vi "ScanFlyCap.vi"() -> ()   [LabVIEW 2022 SP3]
uses:
  <vilib>/userdefined/High Color/IMAQdx.ctl
  <vilib>/Utility/file.llb/Write To Spreadsheet File (DBL).vi
  <vilib>/vision/driver/NI_Vision_Acquisition_Software.lvlib
  <resource>/objmgr/IMAQImage.rc
panel:
  out "Identify":i32
  in  "ActiveFlyCapControl":refnum<k7>(container)
  in  "ExitSendCmd":bool
  out "X":dbl[](array[numeric])
  in  "Tab Control":enum32{"Image", "Scan", "Motors", "Spectra"}(tab)
  out "Camera?":bool
  out "Image":T1(plugin-control)
  out "Remaining Minutes":i32
  out "Progress Bar":dbl(slide) scale=0.0..1.0
  in  "Sample #":u16
  in  "Save Folder":path=path "D:/Scan Test"
  in  "Root File Name":string="Sample"
  out "Cross Plane Length (mm)":sgl=128.0 format="%.3f"
  out "Scan Plane Length (mm)":sgl=128.0 format="%.3f"
  in  "Distance between\nscan lines (mm)":sgl=1.0 min=0.06 max=1000 step=0.06
  in  "Distance between\nplanes (mm)":sgl=1.0 min=0.06 max=1000 step=0.06
  in  "number of planes":u16=1660
  in  "lines per plane":u16=1660 min=1
  out "current plane":u16
  out "current line":u16
  in  "Abort":bool
  in  "start scan":bool
  out "Current File":path
  in  "Axis 2":refnum<k7>(container)
  in  "Axis 1":refnum<k7>(container)
  in  "Home Seq":bool
  in  "Go Home":bool
  out "XY Graph":cluster{"X":dbl[], "Spectral Amplitude":dbl[]}(graph)
  in  "Exposure (*2.375 ms)":u16=2 format="%.3f"
  in  "Display as wavelngth?":bool=TRUE
  in  "Average#":i32=1 min=1
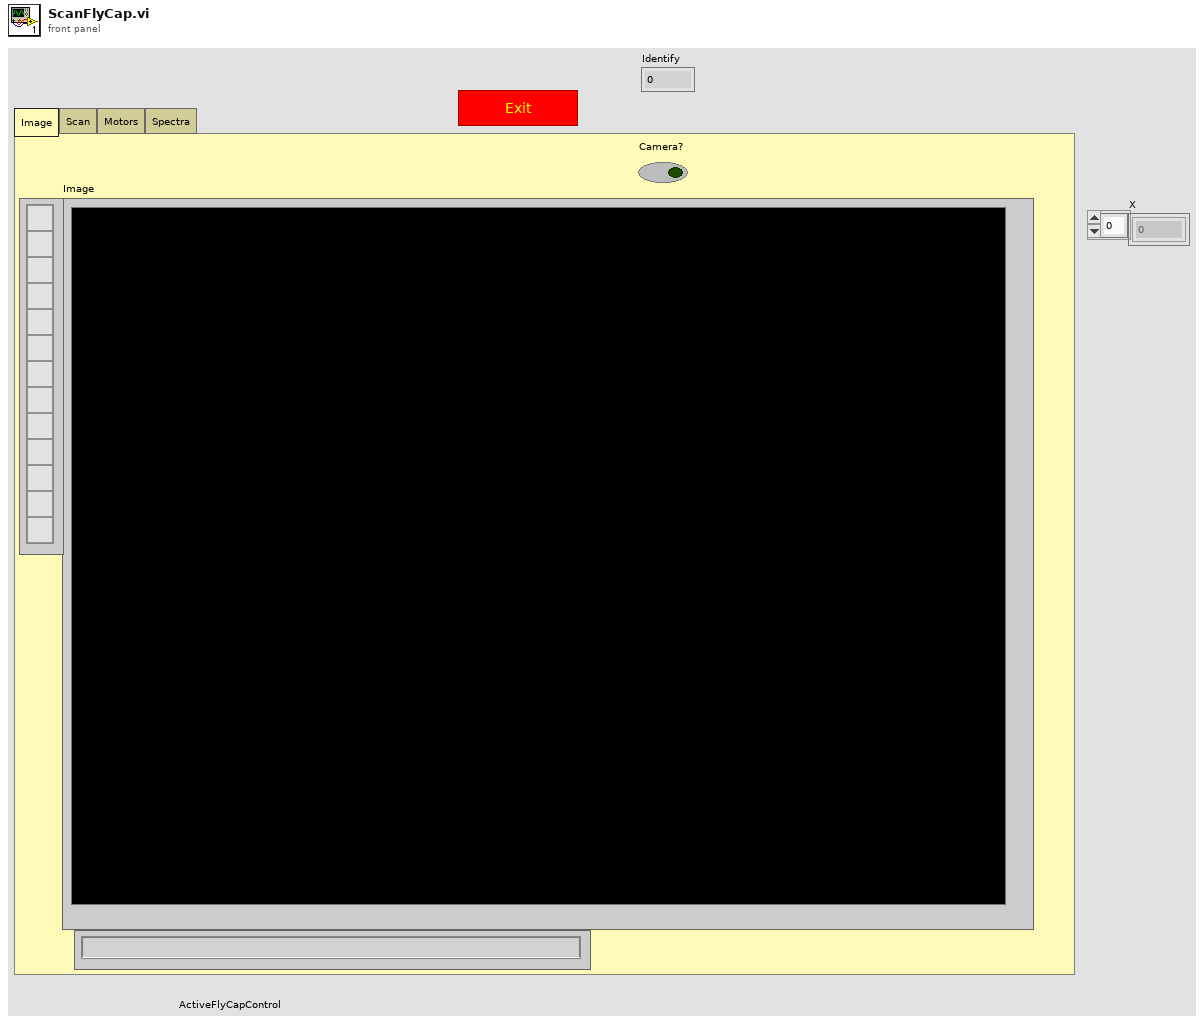
[diagram p1: front panel]
types:
  T1 = typedef "IMAQ Image.ctl" = refnum<image>
  T2 = typedef "Image Type" = u32
  T3 = typedef "IMAQdx.ctl" = refnum<k21>
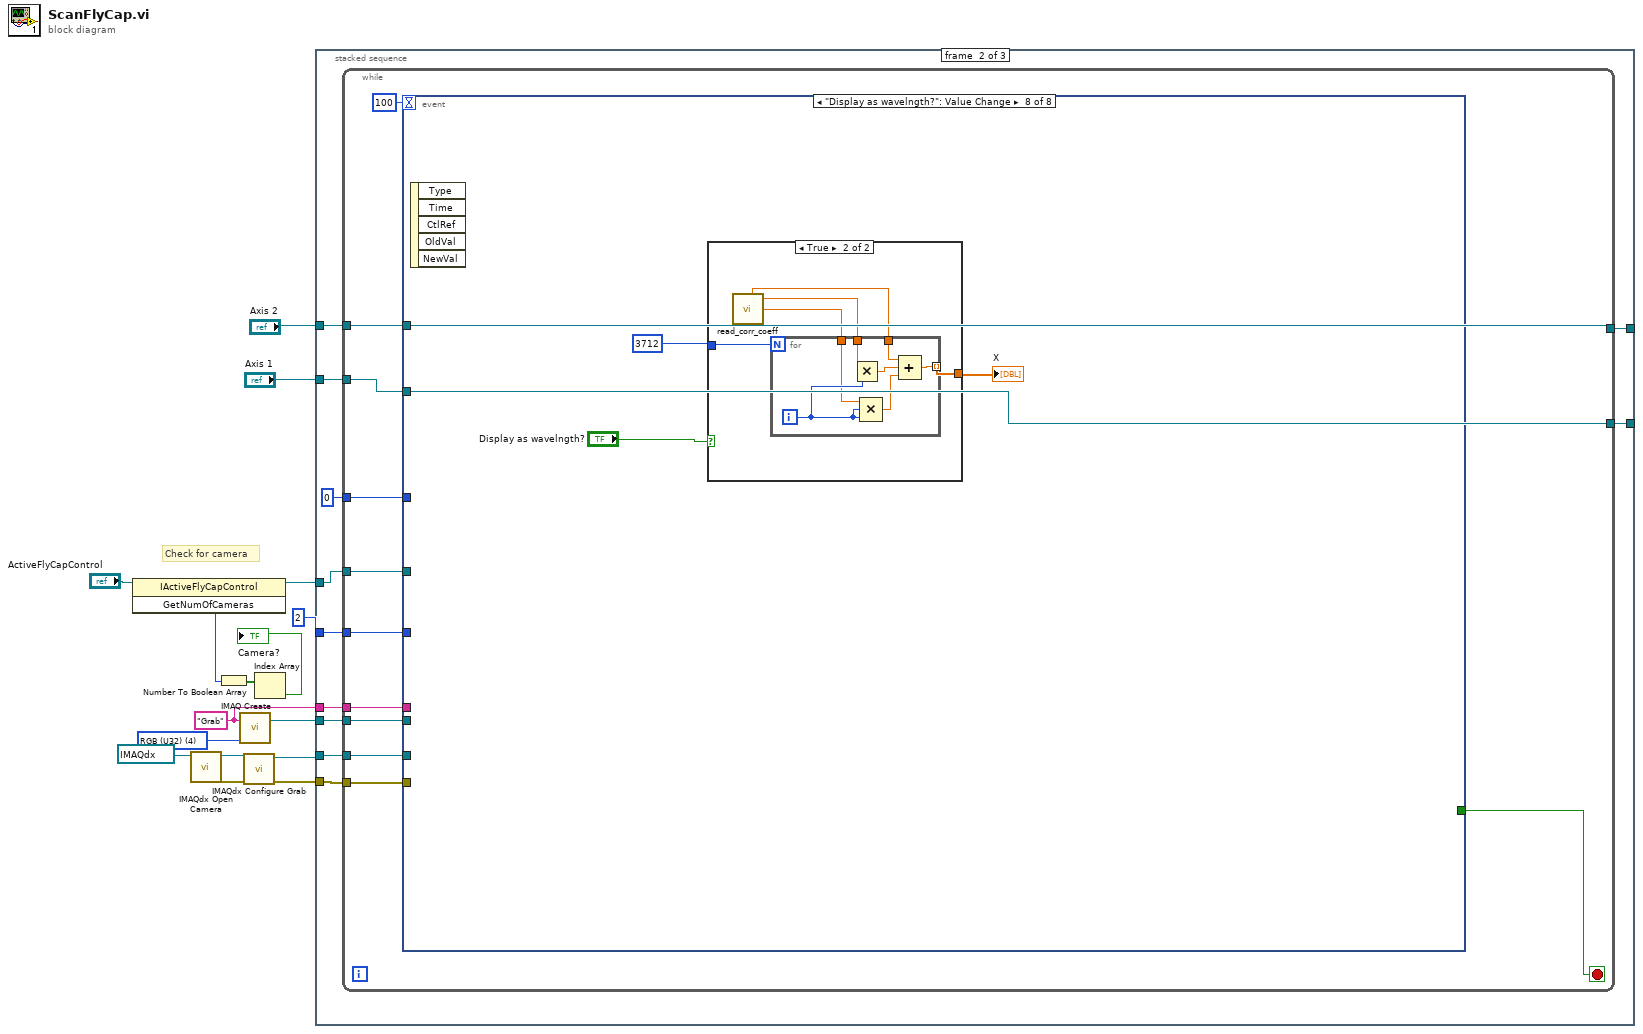
[diagram p0: block diagram]
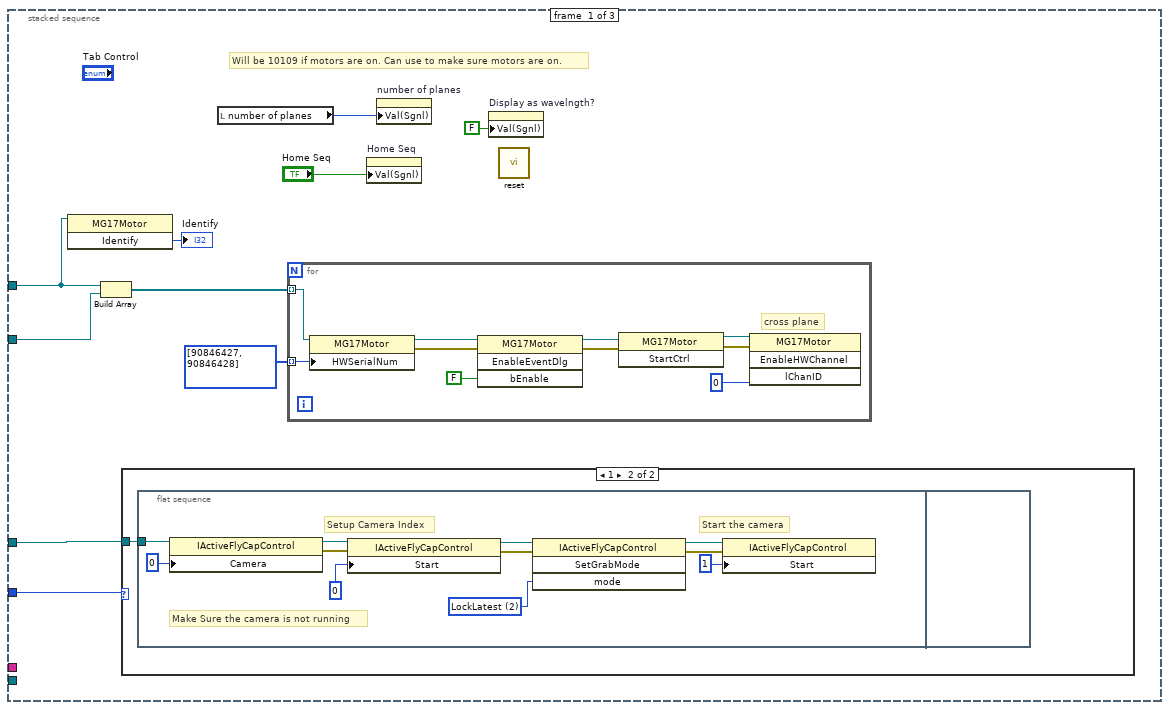
[diagram p2: hidden frame]
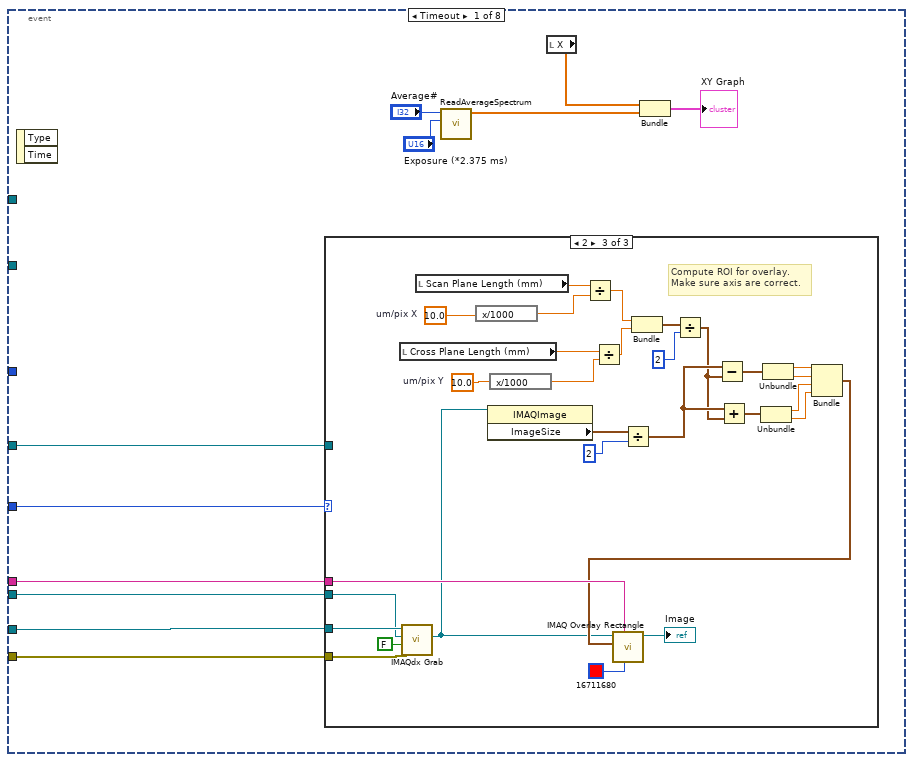
[diagram p4: hidden frame]
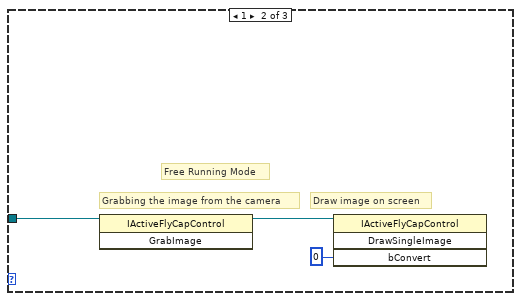
[diagram p6: hidden frame]
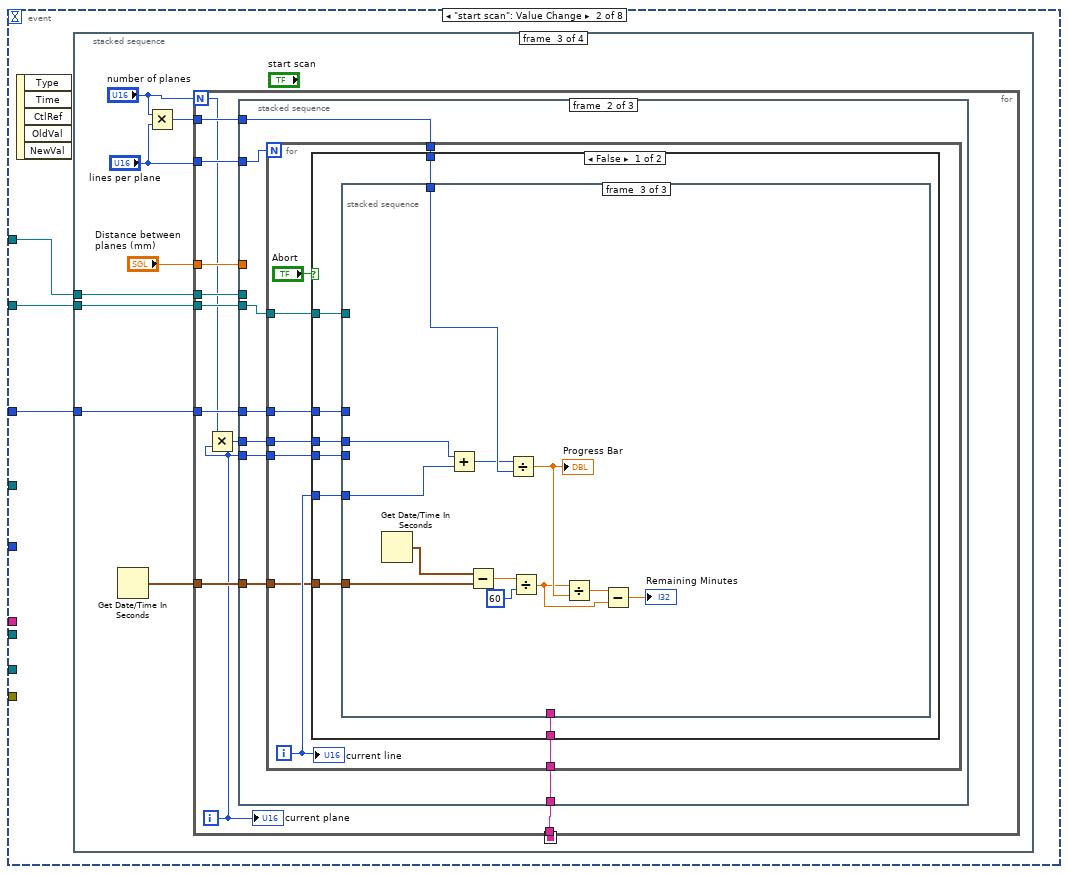
[diagram p7: hidden frame]
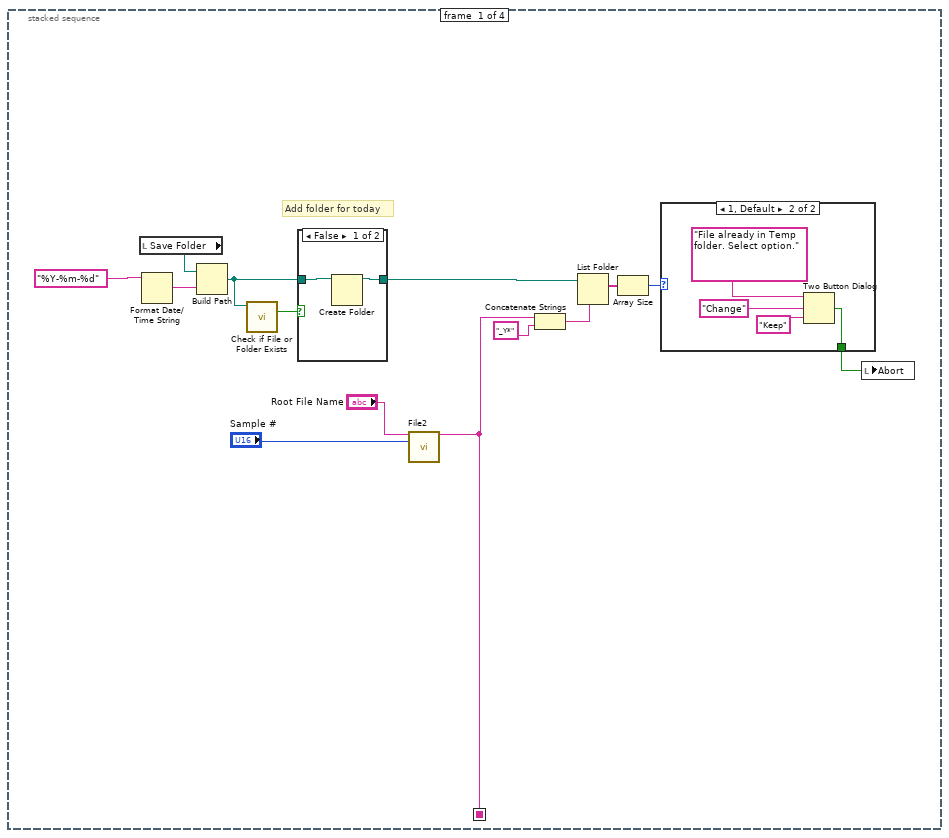
[diagram p8: hidden frame]
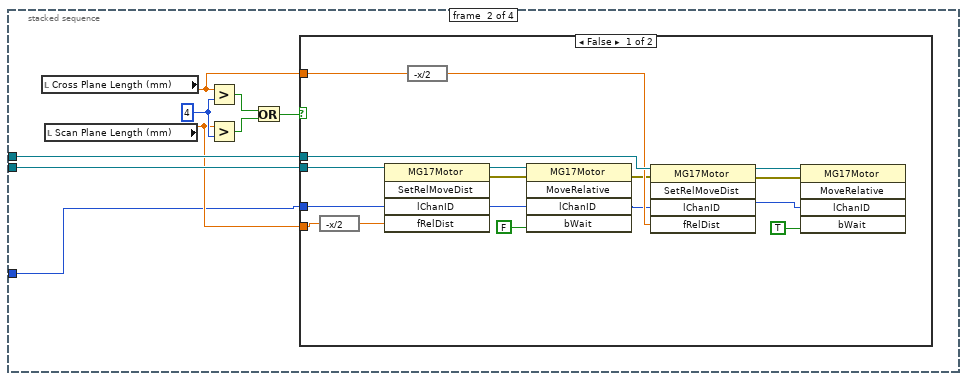
[diagram p11: hidden frame]
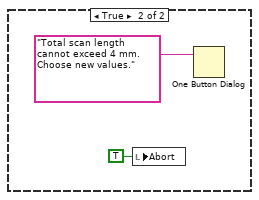
[diagram p12: hidden frame]
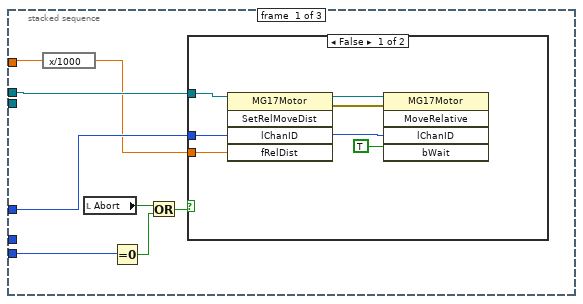
[diagram p13: hidden frame]
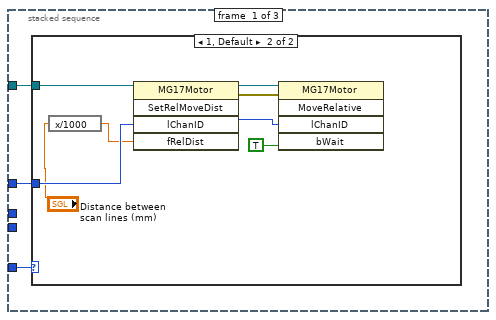
[diagram p15: hidden frame]
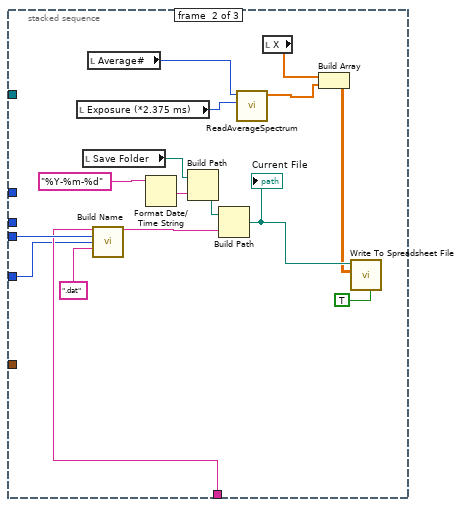
[diagram p17: hidden frame]
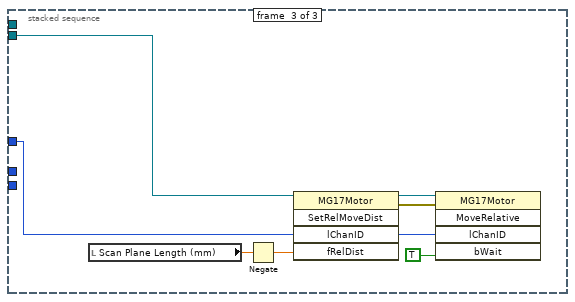
[diagram p19: hidden frame]
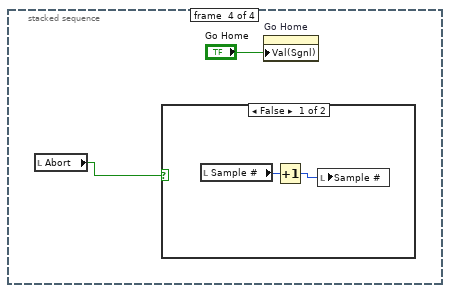
[diagram p20: hidden frame]
diagram:
  w2 = T2 4 items=["Grayscale (U8)", "Grayscale (I16)", "Grayscale (SGL)", "Complex (CSG)", "RGB (U32)", "HSL (U32)", "RGB (U64)", "Grayscale (U16)"] ("Image Type")
  w3 = "Grab" ("Image Name")
  # "Check for camera"
  n1 = invoke class="IActiveFlyCapControl" method="GetNumOfCameras"(reference="ActiveFlyCapControl") -> (reference out=w10:refnum<k7>, "GetNumOfCameras"=w14:i32)  [unwired: 2 in, 1 out]
  n2 = call <vilib>:"IMAQdx Open Camera.vi"("Session In"=T3 "cam0") -> ("error out"=w8:errorcluster, "Session Out"=w9:T3)  [unwired: 2 in, 7 out]
  n3 = Number To Boolean Array(number=w14) -> (Boolean array=w13:bool[])
  n4 = call "IMAQ Create"("Image Name"=w3, "Image Type"=w2) -> ("New Image"=w6:T1)  [unwired: 2 in, 2 out]
  n5 = call <vilib>:"IMAQdx Configure Grab.vi"("error in"=w8, "Session In"=w9) -> ("error out"=w5:errorcluster, "Session Out"=w7:T3)  [unwired: 1 in, 7 out]
  n6 = Index Array(array=w13) -> (element=→"Camera?":bool)  [unwired: 1 in]
  n7 = stacked-sequence {
    tunnel: [_ w58 _] -> _
    tunnel: [_ w57 _] -> _
    tunnel: w10 -> [w21 w56 w381]
    tunnel: 2 ("bConvert") -> [w19 w55 w380]
    tunnel: "Axis 2" -> [w18 w54 w379]
    tunnel: "Axis 1" -> [w20 w53 w378]
    tunnel: w7 -> [_ w52 w376]
    tunnel: w6 -> [_ w51 w377]
    tunnel: w5 -> [_ w49 w375]
    tunnel: w3 -> [_ w50 _]
    frame #0 {
      # "Will be 10109 if motors are on. Can use to make sure motors are on."
      n8 = invoke class="MG17Motor" method="Identify"(reference=w18) -> ("Identify"=→"Identify":i32)  [unwired: 2 in, 2 out]
      n9 = Build Array(w18, w20) -> (w22:refnum<k7>[])
      n10 = case shown="1" w19 {
        tunnel: w21 -> [_ w27]
        frame 0, Default {
        }
        frame 1 {
          n11 = flat-sequence {
            tunnel: w27 -> [w28]
            frame #0 {
              w31 = 2 items=["FreeRunning", "LockNext", "LockLatest"] ("mode")
              # "Make Sure the camera is not running"
              # "Setup Camera Index"
              # "Start the camera"
              n12 = property class="IActiveFlyCapControl"(reference=w28, "Camera"=0 ("Start")) -> (reference out=w34:refnum<k7>, error out=w36:errorcluster)  [unwired: 1 in]
              n13 = property class="IActiveFlyCapControl"(reference=w34, error in=w36, "Start"=0 ("Camera")) -> (reference out=w32:refnum<k7>, error out=w33:errorcluster)
              n14 = invoke class="IActiveFlyCapControl" method="SetGrabMode"(reference=w32, error in=w33, "mode"=w31) -> (reference out=w35:refnum<k7>, error out=w37:errorcluster)  [unwired: 1 in, 2 out]
              n15 = property class="IActiveFlyCapControl"(reference=w35, error in=w37, "Start"=1) -> ()  [unwired: 2 out]
            }
            frame #1 {
            }
          }
        }
      }
      n16 = local read "number of planes"() -> (w25:u16)
      n17 = for {
        tunnel: i32[] [90846427, 90846428] -> [w40] mode=indexing
        tunnel: w22 -> [w41] mode=indexing
        # "cross plane"
        n18 = property class="MG17Motor"(reference=w41, "HWSerialNum"=w40) -> (reference out=w39:refnum<k7>, error out=w44:errorcluster)  [unwired: 1 in]
        n19 = invoke class="MG17Motor" method="EnableEventDlg"(reference=w39, error in=w44, "bEnable"=FALSE ("pbCommsOK")) -> (reference out=w43:refnum<k7>, error out=w42:errorcluster)  [unwired: 1 in, 2 out]
        n20 = invoke class="MG17Motor" method="StartCtrl"(reference=w43, error in=w42) -> (reference out=w48:refnum<k7>, error out=w47:errorcluster)  [unwired: 1 in, 1 out]
        n21 = invoke class="MG17Motor" method="EnableHWChannel"(reference=w48, error in=w47, "lChanID"=0) -> ()  [unwired: 1 in, 4 out]
      }
      n22 = property on="Home Seq" class="Bool (strict)"("Val(Sgnl)"="Home Seq") -> ()  [unwired: 2 in, 2 out]
      n23 = property on="number of planes" class="DigNum (strict)"("Val(Sgnl)"=w25) -> ()  [unwired: 2 in, 2 out]
      n24 = property on="Display as wavelngth?" class="Bool (strict)"("Val(Sgnl)"=FALSE ("Value (Signaling)")) -> ()  [unwired: 2 in, 2 out]
      n25 = call "reset.vi"() -> ()  [unwired: 1 in]
    }
    frame #1 {
      n26 = while {
        tunnel: w53 -> [w67]
        tunnel: w54 -> [w68]
        tunnel: 0 ("lChanID") -> [w69]
        tunnel: [w67] -> w58
        tunnel: [w68] -> w57
        tunnel: w56 -> [w65]
        tunnel: w55 -> [w64]
        tunnel: w52 -> [w62]
        tunnel: w51 -> [w63]
        tunnel: w50 -> [w61]
        tunnel: w49 -> [w60]
        stop <- w70 stop-if-true
        n27 = event shown="[7] \"Display as wavelngth?\": Value Change" {
          selector: _ -> [_ _ _ _ _ _ _ _]
          dyn-events: _ -> [_ _ _ _ _ _ _ _]
          timeout: 100 -> [_ _ _ _ _ _ _ _]
          tunnel: w67 -> [_ w114 w287 _ w320 _ _ _]
          tunnel: w68 -> [_ w116 w286 _ w321 _ _ _]
          tunnel: [_ _ _ "ExitSendCmd" _ _ _ _] -> w70
          tunnel: w69 -> [_ w115 w282 _ w317 _ _ _]
          tunnel: w65 -> [w81 _ _ _ _ _ _ _]
          tunnel: w64 -> [w80 _ _ _ _ _ _ _]
          tunnel: w63 -> [w73 _ _ _ _ _ _ _]
          tunnel: w62 -> [w74 _ _ _ _ _ _ _]
          tunnel: w61 -> [w72 _ _ _ _ _ _ _]
          tunnel: w60 -> [w71 _ _ _ _ _ _ _]
          event Timeout {
            n28 = event-data() -> ()  [unwired: 1 in, 2 out]
            n29 = case shown="2" w80 {
              tunnel: w81 -> [_ w83 _]
              tunnel: w74 -> [_ _ w110]
              tunnel: w73 -> [_ _ w107]
              tunnel: w72 -> [_ _ w112]
              tunnel: w71 -> [_ _ w108]
              frame 0, Default {
              }
              frame 1 {
                # "Draw image on screen"
                # "Grabbing the image from the camera"
                # "Free Running Mode"
                n30 = invoke class="IActiveFlyCapControl" method="GrabImage"(reference=w83) -> (reference out=w82:refnum<k7>)  [unwired: 2 in, 2 out]
                n31 = invoke class="IActiveFlyCapControl" method="DrawSingleImage"(reference=w82, "bConvert"=0) -> ()  [unwired: 2 in, 4 out]
              }
              frame 2 {
                w102 = 10.0  # um/pix Y
                w103 = 10.0  # um/pix X
                # "Compute ROI for overlay.\nMake sure axis are correct."
                n32 = local read "Cross Plane Length (mm)"() -> (w86:sgl)
                n33 = call <vilib>:"IMAQdx Grab.vi"("error in"=w108, "Wait for Next Buffer? (Yes)"=FALSE, "Image In"=w107, "Session In"=w110) -> ("Image Out"=w87:T1)  [unwired: 7 out]
                n34 = local read "Scan Plane Length (mm)"() -> (w104:sgl)
                n35 = expression code="x/1000"(w103) -> (w101:dbl)
                n36 = property class="IMAQImage"(reference=w87) -> ("ImageSize"=w106:cluster{"x":i32, "y":i32})  [unwired: 1 in, 2 out]
                n37 = expression code="x/1000"(w102) -> (w85:dbl)
                n38 = Divide(x=w104, y=w101) -> (x/y=w100:dbl)
                n39 = Divide(x=w86, y=w85) -> (x/y=w99:dbl)
                n40 = Divide(x=w106, y=2) -> (x/y=w96:cluster{"x":dbl, "y":dbl})
                n41 = Bundle(w100, w99) -> (w98:cluster{dbl, dbl})  [unwired: 1 in]
                n42 = Divide(x=w98, y=2) -> (x/y=w95:cluster{dbl, dbl})
                n43 = Subtract(x=w96, y=w95) -> (x-y=w94:cluster{dbl, dbl})
                n44 = Add(x=w96, y=w95) -> (x+y=w93:cluster{dbl, dbl})
                n45 = Unbundle(w93) -> (w90:dbl, w89:dbl)
                n46 = Unbundle(w94) -> (w92:dbl, w91:dbl)
                n47 = Bundle(w92, w91, w90, w89) -> (w88:cluster{dbl, dbl, dbl, dbl})  [unwired: 1 in]
                n48 = call "IMAQ Overlay Rectangle"("Color"=u32 16711680, "Group"=w112, "Rectangle"=w88, "Image"=w87) -> ("Image Out"=→"Image":T1)  [unwired: 6 in, 1 out]
              }
            }
            n49 = call "ReadAverageSpectrum.vi"("Exposure (*2.375 ms)"="Exposure (*2.375 ms)", "Average#"="Average#") -> ("Spectral Amplitude"=w75:dbl[])  [unwired: 9 in]
            n50 = local read "X"() -> (w79:dbl[])
            n51 = Bundle("X"=w79, "Spectral Amplitude"=w75) -> (→"XY Graph":cluster{"X":dbl[], "Spectral Amplitude":dbl[]})  [unwired: 1 in]
          }
          event "start scan": Value Change {
            n52 = event-data() -> ()  [unwired: 1 in, 5 out]
            n53 = stacked-sequence {
              seq-local: [w122 _ _ _] -> [_ _ w170 _]
              tunnel: w116 -> [_ w142 w174 _]
              tunnel: w114 -> [_ w143 w172 _]
              tunnel: w115 -> [_ w138 w171 _]
              frame #0 {
                # "Add folder for today"
                n54 = local read "Save Folder"() -> (w124:path)
                n55 = Format Date/Time String(time format string (%c)="%Y-%m-%d") -> (date/time string=w125:string)  [unwired: 2 in]
                n56 = Build Path(base path=w124, name or relative path=w125) -> (appended path=w119:path)
                n57 = call <vilib>:"Check if File or Folder Exists.vi"("path"=w119) -> ("file or folder exists?"=w118:bool)  [unwired: 8 in, 2 out]
                n58 = case shown="False" w118 {
                  tunnel: w119 -> [w136 w137]
                  tunnel: [w135 w137] -> w123
                  frame False {
                    n59 = Create Folder(path (use dialog)=w136) -> (created path=w135:path)  [unwired: 2 in, 2 out]
                  }
                  frame True {
                  }
                }
                n60 = call "File2"("Beginning Text"="Root File Name", "d"="Sample #") -> ("Result"=w122:string)  [unwired: 12 in, 1 out]
                n61 = Concatenate Strings(w122, "_Y*") -> (w130:string)
                n62 = List Folder(path=w123, pattern=w130) -> (filenames=w129:string[])  [unwired: 1 in, 4 out]
                n63 = Array Size(array=w129) -> (size(s)=w128:i32)
                n64 = case shown="1, Default" w128 {
                  tunnel: [_ w131] -> w126
                  frame 0 {
                  }
                  frame 1, Default {
                    n65 = Two Button Dialog(message="File already in Temp folder. Select option.", 1:"Keep" ("F button name (\"Cancel\")"), 2:"Change" ("T button name (\"OK\")")) -> (T button?=w131:bool)
                  }
                }
                n66 = local write "Abort"(w126) -> ()
              }
              frame #1 {
                w145 = 4
                n67 = local read "Cross Plane Length (mm)"() -> (w141:sgl)
                n68 = local read "Scan Plane Length (mm)"() -> (w140:sgl)
                n69 = Greater?(x=w141, y=w145) -> (0:w146:bool)
                n70 = Greater?(x=w140, y=w145) -> (0:w144:bool)
                n71 = Or(x=w146, y=w144) -> (x .or. y?=w139:bool)
                n72 = case shown="False" w139 {
                  tunnel: w143 -> [w157 _]
                  tunnel: w142 -> [w156 _]
                  tunnel: w138 -> [w151 _]
                  tunnel: w141 -> [w155 _]
                  tunnel: w140 -> [w154 _]
                  frame False {
                    n73 = expression code="-x/2"(w154) -> (w153:sgl)
                    n74 = invoke class="MG17Motor" method="SetRelMoveDist"(reference=w157, "lChanID"=w151, "fRelDist"=w153) -> (reference out=w162:refnum<k7>, error out=w148:errorcluster, "lChanID"=w161:i32)  [unwired: 2 in, 2 out]
                    n75 = expression code="-x/2"(w155) -> (w152:sgl)
                    n76 = invoke class="MG17Motor" method="MoveRelative"(reference=w162, error in=w148, "lChanID"=w161, "bWait"=FALSE) -> (error out=w149:errorcluster, "lChanID"=w147:i32)  [unwired: 1 in, 3 out]
                    n77 = invoke class="MG17Motor" method="SetRelMoveDist"(reference=w156, error in=w149, "lChanID"=w147, "fRelDist"=w152) -> (reference out=w159:refnum<k7>, error out=w150:errorcluster, "lChanID"=w158:i32)  [unwired: 1 in, 2 out]
                    n78 = invoke class="MG17Motor" method="MoveRelative"(reference=w159, error in=w150, "lChanID"=w158, "bWait"=TRUE) -> ()  [unwired: 1 in, 5 out]
                  }
                  frame True {
                    n79 = local write "Abort"(TRUE ("Abort")) -> ()
                    n80 = One Button Dialog(message="Total scan length cannot exceed 4 mm. Choose new values.") -> ()  [unwired: 1 in, 1 out]
                  }
                }
              }
              frame #2 {
                n81 = Get Date/Time In Seconds() -> (seconds since 1Jan1904=w166:timestamp)
                n82 = Multiply(x="number of planes", y="lines per plane") -> (x*y=w167:u16)
                n83 = for {
                  N: "number of planes" -> [w177]
                  tunnel: "lines per plane" -> [w185]
                  tunnel: w174 -> [w184]
                  tunnel: "Distance between\nplanes (mm)" -> [w183]
                  tunnel: w172 -> [w182]
                  tunnel: w171 -> [w181]
                  tunnel: w170 -> [w180]
                  tunnel: w167 -> [w179]
                  tunnel: w166 -> [w178]
                  i -> [w176]
                  n84 = Multiply(x=w177, y=w176) -> (x*y=w175:i32)
                  n85 = stacked-sequence {
                    tunnel: w185 -> [_ w208 _]
                    tunnel: w184 -> [w193 _ _]
                    tunnel: w183 -> [w191 _ _]
                    tunnel: w182 -> [_ w207 w266]
                    tunnel: w181 -> [w192 w206 w267]
                    tunnel: w176 -> [w186 w205 _]
                    tunnel: w180 -> [_ w204 _]
                    tunnel: w179 -> [_ w203 _]
                    tunnel: w178 -> [_ w202 _]
                    tunnel: w175 -> [_ w201 _]
                    frame #0 {
                      n86 = expression code="x/1000"(w191) -> (w190:sgl)
                      n87 = local read "Abort"() -> (w189:bool)
                      n88 = Equal To 0?(x=w186) -> (x = 0?=w188:bool)
                      n89 = Or(x=w189, y=w188) -> (x .or. y?=w187:bool)
                      n90 = case shown="False" w187 {
                        tunnel: w193 -> [w199 _]
                        tunnel: w192 -> [w196 _]
                        tunnel: w190 -> [w195 _]
                        frame False {
                          n91 = invoke class="MG17Motor" method="SetRelMoveDist"(reference=w199, "lChanID"=w196, "fRelDist"=w195) -> (reference out=w198:refnum<k7>, error out=w194:errorcluster, "lChanID"=w197:i32)  [unwired: 2 in, 2 out]
                          n92 = invoke class="MG17Motor" method="MoveRelative"(reference=w198, error in=w194, "lChanID"=w197, "bWait"=TRUE) -> ()  [unwired: 1 in, 5 out]
                        }
                        frame True {
                        }
                      }
                    }
                    frame #1 {
                      n93 = for {
                        N: w208 -> [_]
                        tunnel: w207 -> [w217]
                        tunnel: w206 -> [w216]
                        tunnel: w205 -> [w213]
                        tunnel: w204 -> [w212]
                        tunnel: w203 -> [w211]
                        tunnel: w202 -> [w210]
                        tunnel: w201 -> [w209]
                        i -> [w214]
                        n94 = case shown="False" "Abort" {
                          tunnel: w217 -> [w225 _]
                          tunnel: w216 -> [w224 _]
                          tunnel: w214 -> [w223 _]
                          tunnel: w213 -> [w222 _]
                          tunnel: w212 -> [w221 _]
                          tunnel: w211 -> [w220 _]
                          tunnel: w210 -> [w219 _]
                          tunnel: w209 -> [w218 _]
                          frame False {
                            n95 = stacked-sequence {
                              tunnel: w225 -> [w228 _ _]
                              tunnel: w224 -> [w227 _ _]
                              tunnel: w223 -> [w226 w248 w263]
                              tunnel: w222 -> [_ w252 _]
                              tunnel: w221 -> [_ w251 _]
                              tunnel: w220 -> [_ _ w264]
                              tunnel: w219 -> [_ _ w260]
                              tunnel: w218 -> [_ _ w261]
                              frame #0 {
                                n96 = case shown="1, Default" w226 {
                                tunnel: w228 -> [_ w233]
                                tunnel: w227 -> [_ w232]
                                frame 0 {
                                }
                                frame 1, Default {
                                n97 = expression code="x/1000"("Distance between\nscan lines (mm)") -> (w230:sgl)
                                n98 = invoke class="MG17Motor" method="SetRelMoveDist"(reference=w233, "lChanID"=w232, "fRelDist"=w230) -> (reference out=w235:refnum<k7>, error out=w231:errorcluster, "lChanID"=w234:i32)  [unwired: 2 in, 2 out]
                                n99 = invoke class="MG17Motor" method="MoveRelative"(reference=w235, error in=w231, "lChanID"=w234, "bWait"=TRUE) -> ()  [unwired: 1 in, 5 out]
                                }
                                }
                              }
                              frame #1 {
                                n100 = local read "Exposure (*2.375 ms)"() -> (w241:u16)
                                n101 = local read "Save Folder"() -> (w238:path)
                                n102 = local read "Average#"() -> (w242:i32)
                                n103 = call "Build Name"("Beginning Text"=w251, "plane"=w252, "line"=w248, "file_EXT"=".dat") -> ("Result"=w247:string)  [unwired: 10 in, 1 out]
                                n104 = Format Date/Time String(time format string (%c)="%Y-%m-%d") -> (date/time string=w240:string)  [unwired: 2 in]
                                n105 = Build Path(base path=w238, name or relative path=w240) -> (appended path=w237:path)
                                n106 = Build Path(base path=w237, name or relative path=w247) -> (appended path=w250:path)
                                "Current File" <- w250
                                n107 = call "ReadAverageSpectrum.vi"("Exposure (*2.375 ms)"=w241, "Average#"=w242) -> ("Spectral Amplitude"=w245:dbl[])  [unwired: 9 in]
                                n108 = local read "X"() -> (w246:dbl[])
                                n109 = Build Array(w246, w245) -> (w244:dbl[][])
                                n110 = call-poly <vilib>:"Write To Spreadsheet File.vi"("transpose? (no:F)"=TRUE, "2D data"=w244, "file path (dialog if empty)"=w250) -> ()  [unwired: 5 in, 1 out]
                              }
                              frame #2 {
                                n111 = Get Date/Time In Seconds() -> (seconds since 1Jan1904=w259:timestamp)
                                n112 = Add(x=w261, y=w263) -> (x+y=w262:i32)
                                n113 = Subtract(x=w259, y=w260) -> (x-y=w258:dbl)
                                n114 = Divide(x=w262, y=w264) -> (x/y=w256:dbl)
                                "Progress Bar" <- w256
                                n115 = Divide(x=w258, y=60) -> (x/y=w254:dbl)
                                n116 = Divide(x=w254, y=w256) -> (x/y=w255:dbl)
                                n117 = Subtract(x=w255, y=w254) -> (x-y=→"Remaining Minutes":dbl)
                              }
                            }
                          }
                          frame True {
                          }
                        }
                        "current line" <- w214
                      }
                    }
                    frame #2 {
                      n118 = local read "Scan Plane Length (mm)"() -> (w268:sgl)
                      n119 = Negate(x=w268) -> (-x=w265:sgl)
                      n120 = invoke class="MG17Motor" method="SetRelMoveDist"(reference=w266, "lChanID"=w267, "fRelDist"=w265) -> (reference out=w270:refnum<k7>, error out=w272:errorcluster, "lChanID"=w271:i32)  [unwired: 2 in, 2 out]
                      n121 = invoke class="MG17Motor" method="MoveRelative"(reference=w270, error in=w272, "lChanID"=w271, "bWait"=TRUE) -> ()  [unwired: 1 in, 5 out]
                    }
                  }
                  "current plane" <- w176
                }
              }
              frame #3 {
                n122 = local read "Abort"() -> (w273:bool)
                n123 = case shown="False" w273 {
                  frame False {
                    n124 = local read "Sample #"() -> (w275:u16)
                    n125 = Increment(x=w275) -> (x+1=w276:u16)
                    n126 = local write "Sample #"(w276) -> ()
                  }
                  frame True {
                    n127 = local write "Abort"(FALSE ("Abort")) -> ()
                  }
                }
                n128 = property on="Go Home" class="Bool (strict)"("Val(Sgnl)"="Go Home") -> ()  [unwired: 2 in, 2 out]
              }
            }
          }
          event "Home Seq": Value Change {
            n129 = event-data() -> ()  [unwired: 1 in, 5 out]
            n130 = invoke class="MG17Motor" method="GetStatusBits_Bits"(reference=w286, "lChanID"=w282) -> ("GetStatusBits_Bits"=w285:i32)  [unwired: 2 in, 3 out]
            n131 = Number To Boolean Array(number=w285) -> (Boolean array=w284:bool[])
            n132 = Index Array(array=w284, index=10) -> (element=w280:bool)
            n133 = case shown="True" w280 {
              tunnel: [_ w289] -> w279
              frame False {
              }
              frame True {
                n134 = Two Button Dialog(message="Home Sequence Was Already Performed", 1:"Override" ("F button name (\"Cancel\")")) -> (T button?=w289:bool)  [unwired: 1 in]
              }
            }
            n135 = local write "Home Seq"(FALSE ("Home Seq")) -> ()
            n136 = case shown="False" w279 {
              tunnel: w287 -> [w293 w306]
              tunnel: w282 -> [w295 _]
              tunnel: w286 -> [w294 w307]
              frame False {
                n137 = Build Array(w294, w293) -> (w292:refnum<k7>[])
                n138 = for {
                  tunnel: w295 -> [w305]
                  tunnel: w292 -> [w304] mode=indexing
                  tunnel: bool[] [FALSE, TRUE] -> [w303] mode=indexing
                  w301 = sgl 0.5  # pfPitch
                  w298 = 1  # plDirSense
                  w302 = 1  # plUnits
                  n139 = invoke class="MG17Motor" method="MoveHome"(reference=w304, "lChanID"=w305, "bWait"=w303) -> (reference out=w296:refnum<k7>)  [unwired: 2 in, 4 out]
                  n140 = invoke class="MG17Motor" method="SetStageAxisInfo"(reference=w296, "lChanID"=0 ("lLimitMode"), "fMinPos"=sgl 0.0, "fMaxPos"=sgl 4.0, "lUnits"=w302, "fPitch"=w301, "lDirSense"=w298) -> ()  [unwired: 2 in, 9 out]
                }
              }
              frame True {
                n141 = Build Array(w307, w306) -> (w308:refnum<k7>[])
                n142 = for {
                  tunnel: w308 -> [w309] mode=indexing
                  w314 = sgl 0.5  # pfPitch
                  w311 = 1  # plDirSense
                  w315 = 1  # plUnits
                  n143 = invoke class="MG17Motor" method="SetStageAxisInfo"(reference=w309, "lChanID"=0 ("lLimitMode"), "fMinPos"=sgl 0.0, "fMaxPos"=sgl 4.0, "lUnits"=w315, "fPitch"=w314, "lDirSense"=w311) -> ()  [unwired: 2 in, 9 out]
                }
              }
            }
            n144 = property on="Go Home" class="Bool (strict)"("Val(Sgnl)"=FALSE ("Value (Signaling)")) -> ()  [unwired: 2 in, 2 out]
          }
          event "ExitSendCmd": Value Change {
            n145 = event-data() -> ()  [unwired: 1 in, 5 out]
          }
          event "Go Home": Value Change {
            n146 = event-data() -> ()  [unwired: 1 in, 5 out]
            n147 = Build Array(w321, w320) -> (w319:refnum<k7>[])
            n148 = for {
              tunnel: w319 -> [w324] mode=indexing
              tunnel: bool[] [FALSE, TRUE] -> [w325] mode=indexing
              tunnel: w317 -> [w323]
              n149 = invoke class="MG17Motor" method="SetAbsMovePos"(reference=w324, "lChanID"=w323, "fAbsPos"=sgl 2.0) -> (reference out=w328:refnum<k7>, error out=w326:errorcluster, "lChanID"=w327:i32)  [unwired: 2 in, 2 out]
              n150 = invoke class="MG17Motor" method="MoveAbsolute"(reference=w328, error in=w326, "lChanID"=w327, "bWait"=w325) -> ()  [unwired: 1 in, 5 out]
            }
            n151 = local write "Go Home"(FALSE ("Go Home")) -> ()
          }
          event "number of planes", "lines per plane", "Distance between\nscan lines (mm)", "Distance between\nplanes (mm)": Value Change {
            w331 = 4
            n152 = event-data() -> ()  [unwired: 1 in, 5 out]
            n153 = local read "Distance between\nscan lines (mm)"() -> (w342:sgl)
            n154 = local read "Distance between\nplanes (mm)"() -> (w343:sgl)
            n155 = local read "lines per plane"() -> (w336:u16)
            n156 = local read "number of planes"() -> (w337:u16)
            n157 = Decrement(x=w336) -> (x-1=w340:u16)
            n158 = Decrement(x=w337) -> (x-1=w341:u16)
            n159 = Multiply(x=w342, y=w340) -> (x*y=w338:sgl)
            n160 = Multiply(x=w343, y=w341) -> (x*y=w339:sgl)
            n161 = expression code="x/1000"(w339) -> (w335:sgl)
            "Cross Plane Length (mm)" <- w335
            n162 = expression code="x/1000"(w338) -> (w332:sgl)
            "Scan Plane Length (mm)" <- w332
            n163 = Greater?(x=w335, y=w331) -> (0:w334:bool)
            n164 = Greater?(x=w332, y=w331) -> (0:w330:bool)
            n165 = Or(x=w334, y=w330) -> (x .or. y?=w333:bool)
            n166 = case shown="True" w333 {
              frame False {
              }
              frame True {
                n167 = One Button Dialog(message="Total scan length cannot exceed 4 mm. Choose new values.") -> ()  [unwired: 1 in, 1 out]
              }
            }
          }
          event "Sample #": Value Change {
            # "Check if file name exists already."
            n168 = event-data() -> ("NewVal"=w346:u16)  [unwired: 1 in, 4 out]
            n169 = local read "Root File Name"() -> (w347:string)
            n170 = call "File"("Beginning Text"=w347, "d"=w346) -> ("Result"=w345:string)  [unwired: 12 in, 1 out]
            n171 = Format Date/Time String(time format string (%c)="%Y-%m-%d") -> (date/time string=w350:string)  [unwired: 2 in]
            n172 = Build Path(base path="Save Folder", name or relative path=w350) -> (appended path=w349:path)
            n173 = Concatenate Strings(w345, "_Y*") -> (w355:string)
            n174 = List Folder(path=w349, pattern=w355) -> (filenames=w354:string[])  [unwired: 1 in, 4 out]
            n175 = Array Size(array=w354) -> (size(s)=w348:i32)
            n176 = case shown="1, Default" w348 {
              frame 0 {
              }
              frame 1, Default {
                n177 = One Button Dialog(message="File has been used already. Select a new file name.") -> ()  [unwired: 1 in, 1 out]
              }
            }
          }
          event "Display as wavelngth?": Value Change {
            n178 = event-data() -> ()  [unwired: 1 in, 5 out]
            n179 = case shown="True" "Display as wavelngth?" {
              tunnel: u16 3712 -> [w361 w366]
              tunnel: [w360 w367] -> w358
              frame False {
                n180 = for {
                  N: w361 -> [_]
                  tunnel: [w362] -> w360 mode=indexing
                  i -> [w362]
                }
              }
              frame True {
                n181 = call "read_corr_coeff.vi"() -> ("A\n(Ax^2+Bx+C)"=w363:dbl, "B\n(Ax^2+Bx+C)"=w364:dbl, "C\n(Ax^2+Bx+C)"=w365:dbl)  [unwired: 1 in, 2 out]
                n182 = for {
                  N: w366 -> [_]
                  tunnel: w365 -> [w373]
                  tunnel: w364 -> [w372]
                  tunnel: w363 -> [w369]
                  tunnel: [w371] -> w367 mode=indexing
                  i -> [w370]
                  n183 = Multiply(x=w372, y=w370) -> (x*y=w374:dbl)
                  n184 = Compound Arithmetic op=MULTIPLY(w369, w370, w370) -> (w368:dbl)
                  n185 = Compound Arithmetic op=ADD(w373, w374, w368) -> (w371:dbl)
                }
              }
            }
            "X" <- w358
          }
        }
      }
    }
    frame #2 {
      n186 = case shown="2" w380 {
        tunnel: w381 -> [_ w383 _]
        tunnel: w377 -> [_ _ w387]
        tunnel: w376 -> [_ _ w386]
        tunnel: w375 -> [_ _ w385]
        frame 0, Default {
        }
        frame 1 {
          # "Stop the camera"
          n187 = property class="IActiveFlyCapControl"(reference=w383, "Start"=0) -> ()  [unwired: 1 in, 2 out]
        }
        frame 2 {
          n188 = call <vilib>:"IMAQdx Close Camera.vi"("error in"=w385, "Session In"=w386) -> ("error out"=w388:errorcluster)  [unwired: 9 out]
          n189 = call "Imaq Dispose"("Image"=w387, "error in (no error)"=w388) -> ()  [unwired: 4 in, 1 out]
        }
      }
      n190 = case shown="True" TRUE {
        tunnel: w379 -> [_ w390]
        tunnel: w378 -> [_ w389]
        frame False {
        }
        frame True {
          n191 = invoke class="MG17Motor" method="StopCtrl"(reference=w389) -> ()  [unwired: 2 in, 3 out]
          n192 = invoke class="MG17Motor" method="StopCtrl"(reference=w390) -> ()  [unwired: 2 in, 3 out]
        }
      }
    }
  }
